vi "Initialise Mint Motor Controller connection.vi"(4 "error in (no error)":errorcluster, 7 "MintControls5560Lib.MintControllerCtrl":refnum<k7>(container)) -> (0 "error out":errorcluster, 3 "Controller reference out":refnum<k7>)   [LabVIEW 2015]
doc: "Initilises the connection to the Mint Motor Controller via USB. For the ESS BPM Test Rig the Motor controller is an ABB NextMove ESB-2."
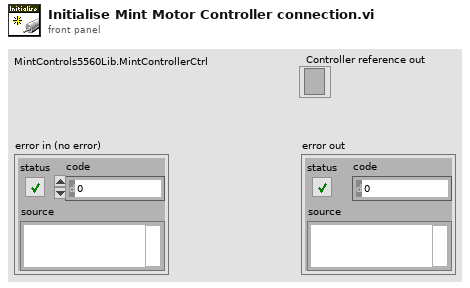
[diagram p1: front panel]
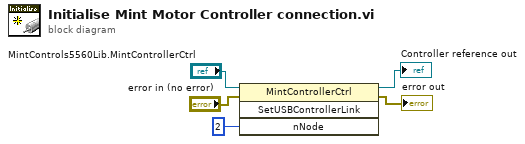
[diagram p0: block diagram]
diagram:
  n1 = invoke class="MintControllerCtrl" method="SetUSBControllerLink"(reference="MintControls5560Lib.MintControllerCtrl", error in="error in (no error)", "nNode"=i16 2) -> (reference out=→"Controller reference out":refnum<k7>, error out=→"error out":errorcluster)  [unwired: 1 in, 2 out]
